vi "Goo03.vi"(10 "ColorSensor":dbl[](array[numeric])=[2.602538796, 2.778320028, 2.755126671, 2.767333701], 11 "클러스터":T1={{"정지할 차이값"=0.08, "흰색과 밖 차이값"=0.15, "흰/검 반 값 "=0.3}, {"4: 오른각도"=122.0, "4: 뒷쪽각도"=0.0, "5: 오른각도"=120.0, "5: 앞쪽각도"=245.0, "6: 왼쪽각도"=245.0, "6: 앞쪽각도"=125.0}, {"2: 공각도"=230.0, "2: 굴릴각도"=60.0}}) -> ()   [LabVIEW 2014]
uses:
  <vilib>/myRIO/Instrument Drivers/Onboard IO/AI/vis/Read.vi
  <vilib>/myRIO/Instrument Drivers/Onboard IO/AI/vis/Smart Open.vi
  <vilib>/Utility/error.llb/Error Cluster From Error Code.vi
  <vilib>/myRIO/Common/Instrument Driver Framework/myRIO v1.0/AI/vis/myRIO v1.0 Read AI.vi
panel:
  in  "第":dbl=500.0
  in  "왼쪽 시간(ms)":u32=680
  in  "뒤로 가는 시간":u32=1100
  out "2: 공각도":u8=230
  in  "Select Servo 2":string(combo)="Servo 2"
  in  "앞으로 갈때 0.6~7초":u32=500
  in  "Select Servo 6":string(combo)="Servo 6"
  in  "Select Servo 5":string(combo)="Servo 5"
  in  "Select Servo 4":string(combo)="Servo 4"
  in  "서브 컨트롤":u8=1
  # "가이드라인 넘어 앞으로간 후, 오른쪽 수평 맞추기"
  # "第: 4"
  # "오: 5"
  # "왼: 6"
  # "190"
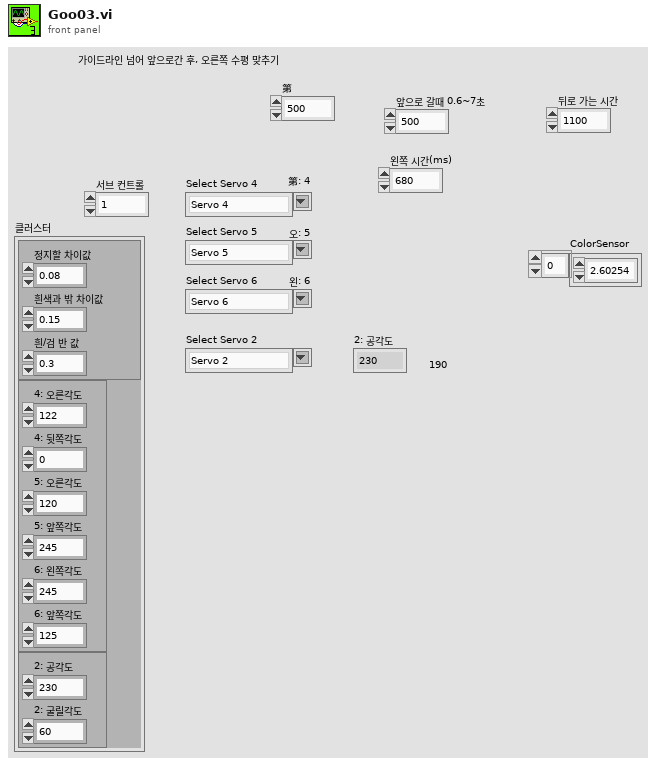
[diagram p1: front panel]
types:
  T1 = cluster{cluster{"정지할 차이값":dbl, "흰색과 밖 차이값":dbl, "흰/검 반 값 ":dbl}, cluster{"4: 오른각도":dbl, "4: 뒷쪽각도":dbl, "5: 오른각도":dbl, "5: 앞쪽각도":dbl, "6: 왼쪽각도":dbl, "6: 앞쪽각도":dbl}, cluster{"2: 공각도":dbl, "2: 굴릴각도":dbl}}
  T2 = cluster{"4: 오른각도":dbl, "4: 뒷쪽각도":dbl, "5: 오른각도":dbl, "5: 앞쪽각도":dbl, "6: 왼쪽각도":dbl, "6: 앞쪽각도":dbl}
  T3 = cluster{"정지할 차이값":dbl, "흰색과 밖 차이값":dbl, "흰/검 반 값 ":dbl}
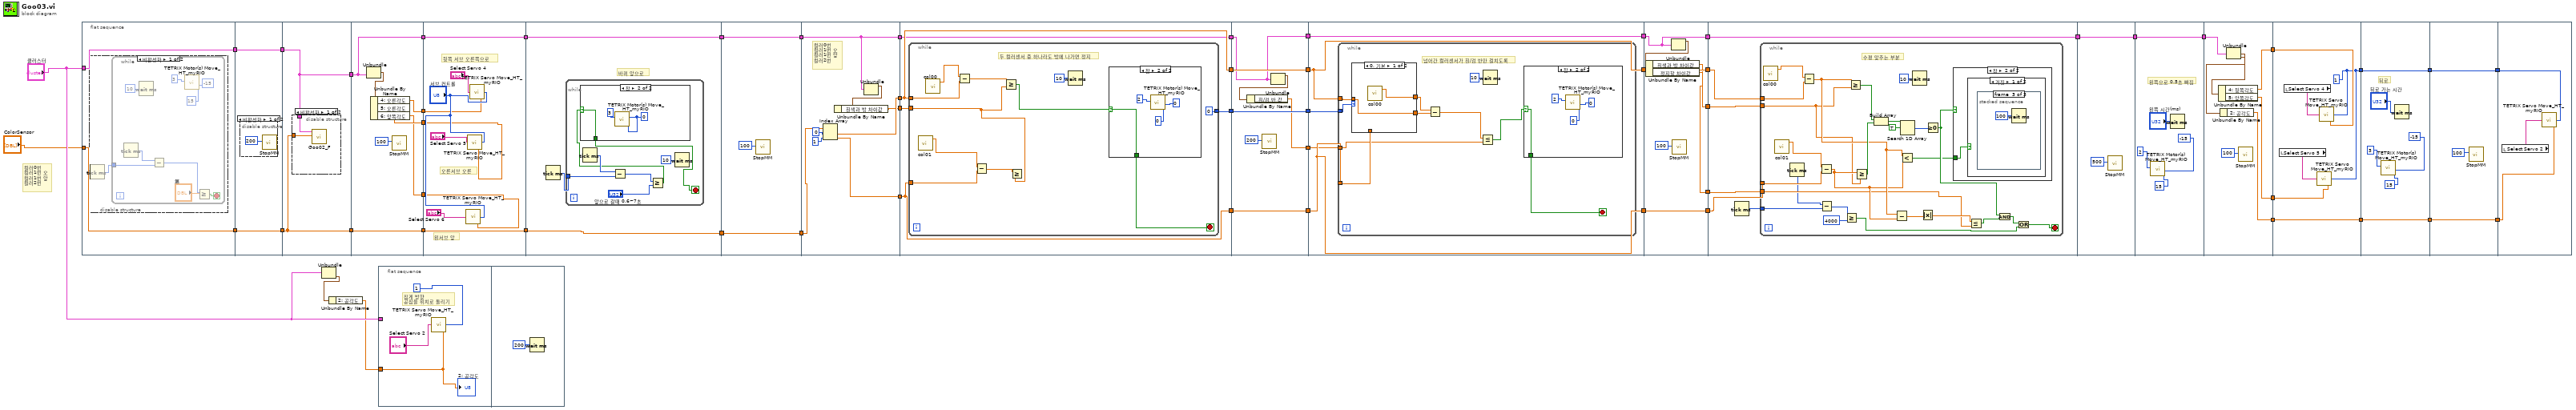
[diagram p0: block diagram]
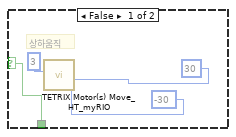
[diagram p5: hidden frame]
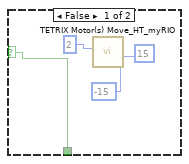
[diagram p6: hidden frame]
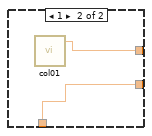
[diagram p7: hidden frame]
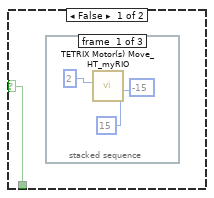
[diagram p8: hidden frame]
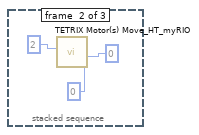
[diagram p9: hidden frame]
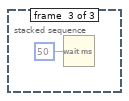
[diagram p10: hidden frame]
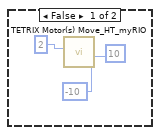
[diagram p11: hidden frame]
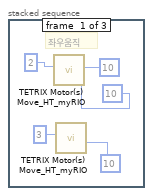
[diagram p12: hidden frame]
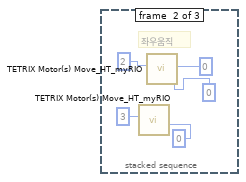
[diagram p13: hidden frame]
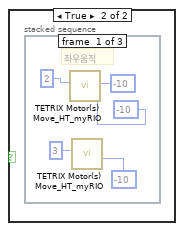
[diagram p14: hidden frame]
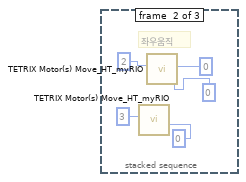
[diagram p15: hidden frame]
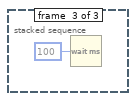
[diagram p16: hidden frame]
diagram:
  # "컬러0번\n컬러1번 오\n컬러1번 앞\n컬러2번"
  n1 = flat-sequence {
    tunnel: "클러스터" -> [w56]
    tunnel: [w56] -> w42
    tunnel: "ColorSensor" -> [w55]
    tunnel: [w55] -> w28
    tunnel: w42 -> [w68]
    tunnel: [w68] -> w41
    tunnel: [w67] -> w29
    tunnel: w28 -> [w67]
    tunnel: w41 -> [w71]
    tunnel: [w71] -> w40
    tunnel: [w70] -> w30
    tunnel: w29 -> [w70]
    tunnel: w40 -> [w74]
    tunnel: [w78] -> w39
    tunnel: [w77] -> w38
    tunnel: [w76] -> w37
    tunnel: [w75] -> w31
    tunnel: w30 -> [w75]
    tunnel: [w74] -> w22
    tunnel: w39 -> [w85]
    tunnel: w38 -> [w84]
    tunnel: w37 -> [w83]
    tunnel: [w82] -> w32
    tunnel: w31 -> [w82]
    tunnel: [w81] -> w23
    tunnel: w22 -> [w81]
    tunnel: w32 -> [w91]
    tunnel: [w91] -> w26
    tunnel: [w90] -> w24
    tunnel: w23 -> [w90]
    tunnel: [w108] -> w27
    tunnel: w26 -> [w108]
    tunnel: [w107] -> w25
    tunnel: w24 -> [w107]
    tunnel: [w115] -> w54
    tunnel: [w113] -> w53
    tunnel: w27 -> [w117]
    tunnel: w25 -> [w112]
    tunnel: [w112] -> w21
    tunnel: [w110] -> w20
    tunnel: w54 -> [w121]
    tunnel: w53 -> [w122]
    tunnel: [w122] -> w52
    tunnel: [w121] -> w51
    tunnel: [w120] -> w43
    tunnel: w21 -> [w118]
    tunnel: w20 -> [w119]
    tunnel: [w118] -> w19
    tunnel: w52 -> [w147]
    tunnel: w51 -> [w148]
    tunnel: [w148] -> w50
    tunnel: [w147] -> w49
    tunnel: [w146] -> w44
    tunnel: w43 -> [w146]
    tunnel: w19 -> [w142]
    tunnel: [w143] -> w18
    tunnel: [w142] -> w16
    tunnel: w50 -> [w153]
    tunnel: [w153] -> w48
    tunnel: w49 -> [w152]
    tunnel: [w152] -> w46
    tunnel: w44 -> [w151]
    tunnel: w18 -> [w150]
    tunnel: [w149] -> w17
    tunnel: w16 -> [w149]
    tunnel: w48 -> [w186]
    tunnel: [w186] -> w47
    tunnel: w46 -> [w185]
    tunnel: [w185] -> w45
    tunnel: w17 -> [w180]
    tunnel: [w182] -> w15
    tunnel: [w181] -> w14
    tunnel: [w180] -> w10
    tunnel: w47 -> [w192]
    tunnel: w45 -> [w191]
    tunnel: w15 -> [w190]
    tunnel: w14 -> [w189]
    tunnel: [w188] -> w11
    tunnel: w10 -> [w188]
    tunnel: [w245] -> w12
    tunnel: w11 -> [w245]
    tunnel: [w247] -> w13
    tunnel: w12 -> [w247]
    tunnel: w13 -> [w257]
    tunnel: [w255] -> w9
    tunnel: [w254] -> w8
    tunnel: [w252] -> w4
    tunnel: w9 -> [w262]
    tunnel: w8 -> [w261]
    tunnel: [w260] -> w5
    tunnel: w4 -> [w260]
    tunnel: [w259] -> w1
    tunnel: [w266] -> w6
    tunnel: w5 -> [w266]
    tunnel: [w265] -> w2
    tunnel: w1 -> [w265]
    tunnel: [w272] -> w7
    tunnel: w6 -> [w272]
    tunnel: [w271] -> w3
    tunnel: w2 -> [w271]
    tunnel: w7 -> [w275]
    tunnel: w3 -> [w274]
    frame #0 {
      n2 = disable-structure shown="비활성화" {
        frame Disabled {
          n3 = Tick Count (ms)() -> (millisecond timer value=w57:u32)
          n4 = while {
            tunnel: w57 -> [w59]
            stop <- w62 stop-if-true
            n5 = Tick Count (ms)() -> (millisecond timer value=w60:u32)
            n6 = Wait (ms)(milliseconds to wait=u32 10 ("대기 시간(ms)")) -> ()  [unwired: 1 out]
            n7 = Subtract(x=w60, y=w59) -> (x-y=w58:u32)
            n8 = call <vilib>:"TETRIX Motor(s) Move_HT_myRIO.vi"("Motor 2 Power (-100 to 100)\n0 = Stop/Brake\n-128 = Stop/Coast"=i8 15 ("Motor 2 Power (-100 to 100)\n0 = Stop/Brake\n-128 = Stop/Coast"), "Motor 1 Power (-100 to 100)\n0 = Stop/Brake\n-128 = Stop/Coast"=i8 -15 ("Motor 1 Power (-100 to 100)\n0 = Stop/Brake\n-128 = Stop/Coast"), "Controller Daisy Chain Position: 1 - 4"=u8 3) -> ()  [unwired: 6 in, 1 out]
            n9 = Greater Or Equal?(x=w58, y="第") -> (x >= y?=w62:bool)
          }
        }
        frame Enabled {
        }
      }
    }
    frame #1 {
      n10 = disable-structure shown="비활성화" {
        frame Disabled {
          n11 = call "StopMM.vi"("대기 시간(ms)"=u32 200) -> ()  [unwired: 11 in]
        }
        frame Enabled {
        }
      }
    }
    frame #2 {
      n12 = disable-structure shown="비활성화" {
        disable-tunnel: w71 -> [w73 _]
        disable-tunnel: w70 -> [w72 _]
        frame Disabled {
          n13 = call "Goo02_F.vi"("ColorSensor 2"=w72, "클러스터"=w73) -> ()  [unwired: 10 in]
        }
        frame Enabled {
        }
      }
    }
    frame #3 {
      n14 = Unbundle(w74) -> (w79:T2)  [unwired: 2 out]
      n15 = Unbundle By Name(w79) -> ("4: 오른각도"=w78:dbl, "5: 오른각도"=w77:dbl, "6: 앞쪽각도"=w76:dbl)
      n16 = call "StopMM.vi"("대기 시간(ms)"=u32 100) -> ()  [unwired: 11 in]
    }
    frame #4 {
      # "왼서브 앞"
      # "오른서브 오른"
      # "뒷쪽 서브 오른쪽으로"
      n17 = call <vilib>:"TETRIX Servo Move_HT_myRIO.vi"("Servo Position (0 - 255)"=w83, "Controller Daisy Chain Position (1 - 4)"="서브 컨트롤", "Select Servo"="Select Servo 6") -> ()  [unwired: 2 in, 1 out]
      n18 = call <vilib>:"TETRIX Servo Move_HT_myRIO.vi"("Servo Position (0 - 255)"=w84, "Controller Daisy Chain Position (1 - 4)"="서브 컨트롤", "Select Servo"="Select Servo 5") -> ()  [unwired: 2 in, 1 out]
      n19 = call <vilib>:"TETRIX Servo Move_HT_myRIO.vi"("Servo Position (0 - 255)"=w85, "Controller Daisy Chain Position (1 - 4)"="서브 컨트롤", "Select Servo"="Select Servo 4") -> ()  [unwired: 2 in, 1 out]
    }
    frame #5 {
      # "바퀴 앞으로"
      n20 = Tick Count (ms)() -> (millisecond timer value=w92:u32)
      n21 = while {
        tunnel: w92 -> [w98]
        stop <- w94 stop-if-true
        n22 = Tick Count (ms)() -> (millisecond timer value=w99:u32)
        n23 = Subtract(x=w99, y=w98) -> (x-y=w97:u32)
        n24 = Greater Or Equal?(x=w97, y="앞으로 갈때 0.6~7초") -> (x >= y?=w93:bool)
        n25 = case shown="참" w93 {
          selector: w93 -> [w100 w106]
          tunnel: [w100 w106] -> w94
          frame False {
            # "상하움직"
            n26 = call <vilib>:"TETRIX Motor(s) Move_HT_myRIO.vi"("Motor 2 Power (-100 to 100)\n0 = Stop/Brake\n-128 = Stop/Coast"=i8 -30 ("Motor 2 Power (-100 to 100)\n0 = Stop/Brake\n-128 = Stop/Coast"), "Motor 1 Power (-100 to 100)\n0 = Stop/Brake\n-128 = Stop/Coast"=i8 30 ("Motor 1 Power (-100 to 100)\n0 = Stop/Brake\n-128 = Stop/Coast"), "Controller Daisy Chain Position: 1 - 4"=u8 3) -> ()  [unwired: 6 in, 1 out]
          }
          frame True {
            w104 = i8 0 ("Motor 1 Power (-100 to 100)\n0 = Stop/Brake\n-128 = Stop/Coast")
            n27 = call <vilib>:"TETRIX Motor(s) Move_HT_myRIO.vi"("Motor 2 Power (-100 to 100)\n0 = Stop/Brake\n-128 = Stop/Coast"=w104, "Motor 1 Power (-100 to 100)\n0 = Stop/Brake\n-128 = Stop/Coast"=w104, "Controller Daisy Chain Position: 1 - 4"=u8 3) -> ()  [unwired: 6 in, 1 out]
          }
        }
        n28 = Wait (ms)(milliseconds to wait=u32 10 ("대기 시간(ms)")) -> ()  [unwired: 1 out]
      }
    }
    frame #6 {
      n29 = call "StopMM.vi"("대기 시간(ms)"=u32 100) -> ()  [unwired: 11 in]
    }
    frame #7 {
      # "컬러0번\n컬러1번 오\n컬러1번 앞\n컬러2번"
      n30 = Index Array(array=w117, index #1=0 ("인덱스"), index #2=1 ("인덱스")) -> (element #1=w115:dbl, element #2=w113:dbl)
      n31 = Unbundle(w112) -> (w111:T3)  [unwired: 2 out]
      n32 = Unbundle By Name(w111) -> ("흰색과 밖 차이값"=w110:dbl)
    }
    frame #8 {
      n33 = while {
        tunnel: w122 -> [w133]
        tunnel: w121 -> [w132]
        tunnel: [0 ("index of element")] -> w120
        tunnel: w119 -> [w126]
        stop <- w123 stop-if-true
        # "두 컬러센서 중 하나라도 밖에 나가면 정지"
        n34 = call "col01.vi"() -> ("Col01 (B/AI1 (Pin 5))"=w124:dbl)  [unwired: 26 in, 1 out]
        n35 = call "col00.vi"() -> ("Col00 (B/AI0 (Pin 3))"=w125:dbl)  [unwired: 26 in, 1 out]
        n36 = Subtract(x=w125, y=w132) -> (x-y=w131:dbl)
        n37 = Subtract(x=w124, y=w133) -> (x-y=w130:dbl)
        n38 = Greater Or Equal?(x=w131, y=w126) -> (x >= y?=w127:bool)
        n39 = Greater Or Equal?(x=w130, y=w126) -> ()  [unwired: 1 out]
        n40 = Wait (ms)(milliseconds to wait=u32 10 ("대기 시간(ms)")) -> ()  [unwired: 1 out]
        n41 = case shown="참" w127 {
          selector: w127 -> [w134 w138]
          tunnel: [w134 w138] -> w123
          frame False {
            n42 = call <vilib>:"TETRIX Motor(s) Move_HT_myRIO.vi"("Motor 2 Power (-100 to 100)\n0 = Stop/Brake\n-128 = Stop/Coast"=i8 -15 ("Motor 2 Power (-100 to 100)\n0 = Stop/Brake\n-128 = Stop/Coast"), "Motor 1 Power (-100 to 100)\n0 = Stop/Brake\n-128 = Stop/Coast"=i8 15 ("Motor 1 Power (-100 to 100)\n0 = Stop/Brake\n-128 = Stop/Coast"), "Controller Daisy Chain Position: 1 - 4"=u8 2) -> ()  [unwired: 6 in, 1 out]
          }
          frame True {
            n43 = call <vilib>:"TETRIX Motor(s) Move_HT_myRIO.vi"("Motor 2 Power (-100 to 100)\n0 = Stop/Brake\n-128 = Stop/Coast"=i8 0 ("Motor 2 Power (-100 to 100)\n0 = Stop/Brake\n-128 = Stop/Coast"), "Motor 1 Power (-100 to 100)\n0 = Stop/Brake\n-128 = Stop/Coast"=i8 0 ("Motor 1 Power (-100 to 100)\n0 = Stop/Brake\n-128 = Stop/Coast"), "Controller Daisy Chain Position: 1 - 4"=u8 2) -> ()  [unwired: 6 in, 1 out]
          }
        }
      }
    }
    frame #9 {
      n44 = call "StopMM.vi"("대기 시간(ms)"=u32 200) -> ()  [unwired: 11 in]
      n45 = Unbundle(w142) -> (w144:T3)  [unwired: 2 out]
      n46 = Unbundle By Name(w144) -> ("흰/검 반 값"=w143:dbl)
    }
    frame #10 {
      n47 = while {
        tunnel: w152 -> [w159]
        tunnel: w153 -> [w160]
        tunnel: w151 -> [w158]
        tunnel: w150 -> [w154]
        stop <- w157 stop-if-true
        # "넘어간 컬러센서가 흰/검 반만 걸치도록"
        n48 = case shown="0, 기본" w158 {
          tunnel: [w164 w166] -> w163
          tunnel: [w165 w167] -> w161
          tunnel: w160 -> [w165 _]
          tunnel: w159 -> [_ w167]
          frame 0, Default {
            n49 = call "col00.vi"() -> ("Col00 (B/AI0 (Pin 3))"=w164:dbl)  [unwired: 26 in, 1 out]
          }
          frame 1 {
            n50 = call "col01.vi"() -> ("Col01 (B/AI1 (Pin 5))"=w166:dbl)  [unwired: 26 in, 1 out]
          }
        }
        n51 = Subtract(x=w163, y=w161) -> (x-y=w155:dbl)
        n52 = Less Or Equal?(x=w155, y=w154) -> (x <= y?=w156:bool)
        n53 = Wait (ms)(milliseconds to wait=u32 10 ("대기 시간(ms)")) -> ()  [unwired: 1 out]
        n54 = case shown="참" w156 {
          selector: w156 -> [w168 w176]
          tunnel: [w168 w176] -> w157
          frame False {
            n55 = stacked-sequence {
              frame #0 {
                n56 = call <vilib>:"TETRIX Motor(s) Move_HT_myRIO.vi"("Motor 2 Power (-100 to 100)\n0 = Stop/Brake\n-128 = Stop/Coast"=i8 15 ("Motor 2 Power (-100 to 100)\n0 = Stop/Brake\n-128 = Stop/Coast"), "Motor 1 Power (-100 to 100)\n0 = Stop/Brake\n-128 = Stop/Coast"=i8 -15 ("Motor 1 Power (-100 to 100)\n0 = Stop/Brake\n-128 = Stop/Coast"), "Controller Daisy Chain Position: 1 - 4"=u8 2) -> ()  [unwired: 6 in, 1 out]
              }
              frame #1 {
                n57 = call <vilib>:"TETRIX Motor(s) Move_HT_myRIO.vi"("Motor 2 Power (-100 to 100)\n0 = Stop/Brake\n-128 = Stop/Coast"=i8 0 ("Motor 2 Power (-100 to 100)\n0 = Stop/Brake\n-128 = Stop/Coast"), "Motor 1 Power (-100 to 100)\n0 = Stop/Brake\n-128 = Stop/Coast"=i8 0 ("Motor 1 Power (-100 to 100)\n0 = Stop/Brake\n-128 = Stop/Coast"), "Controller Daisy Chain Position: 1 - 4"=u8 2) -> ()  [unwired: 6 in, 1 out]
              }
              frame #2 {
                n58 = Wait (ms)(milliseconds to wait=u32 50 ("대기 시간(ms)")) -> ()  [unwired: 1 out]
              }
            }
          }
          frame True {
            n59 = call <vilib>:"TETRIX Motor(s) Move_HT_myRIO.vi"("Motor 2 Power (-100 to 100)\n0 = Stop/Brake\n-128 = Stop/Coast"=i8 0 ("Motor 2 Power (-100 to 100)\n0 = Stop/Brake\n-128 = Stop/Coast"), "Motor 1 Power (-100 to 100)\n0 = Stop/Brake\n-128 = Stop/Coast"=i8 0 ("Motor 1 Power (-100 to 100)\n0 = Stop/Brake\n-128 = Stop/Coast"), "Controller Daisy Chain Position: 1 - 4"=u8 2) -> ()  [unwired: 6 in, 1 out]
          }
        }
      }
    }
    frame #11 {
      n60 = Unbundle(w180) -> (w183:T3)  [unwired: 2 out]
      n61 = Unbundle By Name(w183) -> ("흰색과 밖 차이값"=w182:dbl, "정지할 차이값"=w181:dbl)
      n62 = call "StopMM.vi"("대기 시간(ms)"=u32 100) -> ()  [unwired: 11 in]
    }
    frame #12 {
      n63 = Tick Count (ms)() -> (millisecond timer value=w187:u32)
      n64 = while {
        tunnel: w191 -> [w218]
        tunnel: w192 -> [w217]
        tunnel: w190 -> [w203]
        tunnel: w189 -> [w202]
        tunnel: w187 -> [w198]
        stop <- w194 stop-if-true
        # "수평 맞추는 부분"
        n65 = call "col00.vi"() -> ("Col00 (B/AI0 (Pin 3))"=w201:dbl)  [unwired: 26 in, 1 out]
        n66 = call "col01.vi"() -> ("Col01 (B/AI1 (Pin 5))"=w200:dbl)  [unwired: 26 in, 1 out]
        n67 = Tick Count (ms)() -> (millisecond timer value=w199:u32)
        n68 = Subtract(x=w201, y=w217) -> (x-y=w206:dbl)
        n69 = Subtract(x=w200, y=w218) -> (x-y=w205:dbl)
        n70 = Subtract(x=w199, y=w198) -> (x-y=w197:u32)
        n71 = Greater Or Equal?(x=w197, y=u32 4000) -> (x >= y?=w193:bool)
        n72 = Greater Or Equal?(x=w206, y=w203) -> (x >= y?=w216:bool)
        n73 = Greater Or Equal?(x=w205, y=w203) -> (x >= y?=w215:bool)
        n74 = Build Array(w216, w215) -> (w214:bool[])
        n75 = Subtract(x=w206, y=w205) -> (x-y=w209:dbl)
        n76 = Search 1D Array(1D array=w214, element=TRUE ("원소")) -> (index of element=w212:i32)  [unwired: 1 in]
        n77 = Less?(x=w206, y=w205) -> (x < y?=w204:bool)
        n78 = Wait (ms)(milliseconds to wait=u32 10 ("대기 시간(ms)")) -> ()  [unwired: 1 out]
        n79 = Absolute Value(x=w209) -> (abs(x)=w208:dbl)
        n80 = Greater Or Equal To 0?(x=w212) -> (x >= 0?=w207:bool)
        n81 = case shown="참" w207 {
          tunnel: w204 -> [_ w222]
          frame False {
            n82 = call <vilib>:"TETRIX Motor(s) Move_HT_myRIO.vi"("Motor 2 Power (-100 to 100)\n0 = Stop/Brake\n-128 = Stop/Coast"=i8 -10 ("Motor 2 Power (-100 to 100)\n0 = Stop/Brake\n-128 = Stop/Coast"), "Motor 1 Power (-100 to 100)\n0 = Stop/Brake\n-128 = Stop/Coast"=i8 10 ("Motor 1 Power (-100 to 100)\n0 = Stop/Brake\n-128 = Stop/Coast"), "Controller Daisy Chain Position: 1 - 4"=u8 2) -> ()  [unwired: 6 in, 1 out]
          }
          frame True {
            n83 = case shown="거짓" w222 {
              frame False {
                n84 = stacked-sequence {
                  frame #0 {
                    # "좌우움직"
                    n85 = call <vilib>:"TETRIX Motor(s) Move_HT_myRIO.vi"("Motor 2 Power (-100 to 100)\n0 = Stop/Brake\n-128 = Stop/Coast"=i8 10 ("Motor 2 Power (-100 to 100)\n0 = Stop/Brake\n-128 = Stop/Coast"), "Motor 1 Power (-100 to 100)\n0 = Stop/Brake\n-128 = Stop/Coast"=i8 10 ("Motor 1 Power (-100 to 100)\n0 = Stop/Brake\n-128 = Stop/Coast"), "Controller Daisy Chain Position: 1 - 4"=u8 2) -> ()  [unwired: 6 in, 1 out]
                    n86 = call <vilib>:"TETRIX Motor(s) Move_HT_myRIO.vi"("Motor 1 Power (-100 to 100)\n0 = Stop/Brake\n-128 = Stop/Coast"=i8 10 ("Motor 1 Power (-100 to 100)\n0 = Stop/Brake\n-128 = Stop/Coast"), "Controller Daisy Chain Position: 1 - 4"=u8 3) -> ()  [unwired: 7 in, 1 out]
                  }
                  frame #1 {
                    # "좌우움직"
                    n87 = call <vilib>:"TETRIX Motor(s) Move_HT_myRIO.vi"("Motor 1 Power (-100 to 100)\n0 = Stop/Brake\n-128 = Stop/Coast"=i8 0 ("Motor 1 Power (-100 to 100)\n0 = Stop/Brake\n-128 = Stop/Coast"), "Controller Daisy Chain Position: 1 - 4"=u8 3) -> ()  [unwired: 7 in, 1 out]
                    n88 = call <vilib>:"TETRIX Motor(s) Move_HT_myRIO.vi"("Motor 2 Power (-100 to 100)\n0 = Stop/Brake\n-128 = Stop/Coast"=i8 0 ("Motor 2 Power (-100 to 100)\n0 = Stop/Brake\n-128 = Stop/Coast"), "Motor 1 Power (-100 to 100)\n0 = Stop/Brake\n-128 = Stop/Coast"=i8 0 ("Motor 1 Power (-100 to 100)\n0 = Stop/Brake\n-128 = Stop/Coast"), "Controller Daisy Chain Position: 1 - 4"=u8 2) -> ()  [unwired: 6 in, 1 out]
                  }
                  frame #2 {
                    n89 = Wait (ms)(milliseconds to wait=u32 100 ("대기 시간(ms)")) -> ()  [unwired: 1 out]
                  }
                }
              }
              frame True {
                n90 = stacked-sequence {
                  frame #0 {
                    # "좌우움직"
                    n91 = call <vilib>:"TETRIX Motor(s) Move_HT_myRIO.vi"("Motor 2 Power (-100 to 100)\n0 = Stop/Brake\n-128 = Stop/Coast"=i8 -10 ("Motor 2 Power (-100 to 100)\n0 = Stop/Brake\n-128 = Stop/Coast"), "Motor 1 Power (-100 to 100)\n0 = Stop/Brake\n-128 = Stop/Coast"=i8 -10 ("Motor 1 Power (-100 to 100)\n0 = Stop/Brake\n-128 = Stop/Coast"), "Controller Daisy Chain Position: 1 - 4"=u8 2) -> ()  [unwired: 6 in, 1 out]
                    n92 = call <vilib>:"TETRIX Motor(s) Move_HT_myRIO.vi"("Motor 1 Power (-100 to 100)\n0 = Stop/Brake\n-128 = Stop/Coast"=i8 -10 ("Motor 1 Power (-100 to 100)\n0 = Stop/Brake\n-128 = Stop/Coast"), "Controller Daisy Chain Position: 1 - 4"=u8 3) -> ()  [unwired: 7 in, 1 out]
                  }
                  frame #1 {
                    # "좌우움직"
                    n93 = call <vilib>:"TETRIX Motor(s) Move_HT_myRIO.vi"("Motor 1 Power (-100 to 100)\n0 = Stop/Brake\n-128 = Stop/Coast"=i8 0 ("Motor 1 Power (-100 to 100)\n0 = Stop/Brake\n-128 = Stop/Coast"), "Controller Daisy Chain Position: 1 - 4"=u8 3) -> ()  [unwired: 7 in, 1 out]
                    n94 = call <vilib>:"TETRIX Motor(s) Move_HT_myRIO.vi"("Motor 2 Power (-100 to 100)\n0 = Stop/Brake\n-128 = Stop/Coast"=i8 0 ("Motor 2 Power (-100 to 100)\n0 = Stop/Brake\n-128 = Stop/Coast"), "Motor 1 Power (-100 to 100)\n0 = Stop/Brake\n-128 = Stop/Coast"=i8 0 ("Motor 1 Power (-100 to 100)\n0 = Stop/Brake\n-128 = Stop/Coast"), "Controller Daisy Chain Position: 1 - 4"=u8 2) -> ()  [unwired: 6 in, 1 out]
                  }
                  frame #2 {
                    n95 = Wait (ms)(milliseconds to wait=u32 100 ("대기 시간(ms)")) -> ()  [unwired: 1 out]
                  }
                }
              }
            }
          }
        }
        n96 = Less Or Equal?(x=w208, y=w202) -> (x <= y?=w210:bool)
        n97 = And(x=w207, y=w210) -> (x .and. y?=w195:bool)
        n98 = Or(x=w195, y=w193) -> (x .or. y?=w194:bool)
      }
    }
    frame #13 {
      n99 = call "StopMM.vi"("대기 시간(ms)"=u32 500) -> ()  [unwired: 11 in]
    }
    frame #14 {
      # "왼쪽으로 0.5초 빠짐"
      n100 = call <vilib>:"TETRIX Motor(s) Move_HT_myRIO.vi"("Motor 2 Power (-100 to 100)\n0 = Stop/Brake\n-128 = Stop/Coast"=i8 15 ("Motor 2 Power (-100 to 100)\n0 = Stop/Brake\n-128 = Stop/Coast"), "Motor 1 Power (-100 to 100)\n0 = Stop/Brake\n-128 = Stop/Coast"=i8 -15 ("Motor 1 Power (-100 to 100)\n0 = Stop/Brake\n-128 = Stop/Coast"), "Controller Daisy Chain Position: 1 - 4"=u8 2) -> ()  [unwired: 6 in, 1 out]
      n101 = Wait (ms)(milliseconds to wait="왼쪽 시간(ms)") -> ()  [unwired: 1 out]
    }
    frame #15 {
      n102 = Unbundle(w257) -> (w256:T2, w253:cluster{"2: 공각도":dbl, "2: 굴릴각도":dbl})  [unwired: 1 out]
      n103 = Unbundle By Name(w256) -> ("4: 뒷쪽각도"=w255:dbl, "5: 앞쪽각도"=w254:dbl)
      n104 = Unbundle By Name(w253) -> ("2: 공각도"=w252:dbl)
      n105 = call "StopMM.vi"("대기 시간(ms)"=u32 100) -> ()  [unwired: 11 in]
    }
    frame #16 {
      w259 = u8 1 ("Controller Daisy Chain Position (1 - 4)")
      n106 = local read "Select Servo 5"() -> (w263:string)
      n107 = local read "Select Servo 4"() -> (w264:string)
      n108 = call <vilib>:"TETRIX Servo Move_HT_myRIO.vi"("Servo Position (0 - 255)"=w261, "Controller Daisy Chain Position (1 - 4)"=w259, "Select Servo"=w263) -> ()  [unwired: 2 in, 1 out]
      n109 = call <vilib>:"TETRIX Servo Move_HT_myRIO.vi"("Servo Position (0 - 255)"=w262, "Controller Daisy Chain Position (1 - 4)"=w259, "Select Servo"=w264) -> ()  [unwired: 2 in, 1 out]
    }
    frame #17 {
      # "뒤로"
      n110 = call <vilib>:"TETRIX Motor(s) Move_HT_myRIO.vi"("Motor 2 Power (-100 to 100)\n0 = Stop/Brake\n-128 = Stop/Coast"=i8 15 ("Motor 2 Power (-100 to 100)\n0 = Stop/Brake\n-128 = Stop/Coast"), "Motor 1 Power (-100 to 100)\n0 = Stop/Brake\n-128 = Stop/Coast"=i8 -15 ("Motor 1 Power (-100 to 100)\n0 = Stop/Brake\n-128 = Stop/Coast"), "Controller Daisy Chain Position: 1 - 4"=u8 3) -> ()  [unwired: 6 in, 1 out]
      n111 = Wait (ms)(milliseconds to wait="뒤로 가는 시간") -> ()  [unwired: 1 out]
    }
    frame #18 {
      n112 = call "StopMM.vi"("대기 시간(ms)"=u32 100) -> ()  [unwired: 11 in]
    }
    frame #19 {
      n113 = local read "Select Servo 2"() -> (w276:string)
      n114 = call <vilib>:"TETRIX Servo Move_HT_myRIO.vi"("Servo Position (0 - 255)"=w275, "Controller Daisy Chain Position (1 - 4)"=w274, "Select Servo"=w276) -> ()  [unwired: 2 in, 1 out]
    }
  }
  n115 = Unbundle("클러스터") -> (w35:cluster{"2: 공각도":dbl, "2: 굴릴각도":dbl})  [unwired: 2 out]
  n116 = Unbundle By Name(w35) -> ("2: 공각도"=w34:dbl)
  n117 = flat-sequence {
    tunnel: "클러스터" -> [_]
    tunnel: w34 -> [w278]
    frame #0 {
      # "집게 방향\n공집을 위치로 돌리기"
      n118 = call <vilib>:"TETRIX Servo Move_HT_myRIO.vi"("Servo Position (0 - 255)"=w278, "Controller Daisy Chain Position (1 - 4)"=u8 1, "Select Servo"="Select Servo 2") -> ()  [unwired: 2 in, 1 out]
      "2: 공각도" <- w278
    }
    frame #1 {
      n119 = Wait (ms)(milliseconds to wait=u32 200 ("대기 시간(ms)")) -> ()  [unwired: 1 out]
    }
  }
